vi "read from wavemeter_PB.vi"(2 "error in (no error)":errorcluster, 3 "Single Measurement?":bool=TRUE, 4 "Select Port":refnum<visa-resource-name>="COM1") -> (0 "error out":errorcluster={"status"=FALSE, "code"=1073676294, "source"="VISA Read in read from wavemeter.vi"}, 1 "frequency":string, 5 "Units":string)   [LabVIEW 2013]
uses:
  <vilib>/Instr/_visa.llb/VISA Configure Serial Port (Instr).vi
panel:
  in  "Case Constant\n(See Context Help)":bool
  in  "Tab Control":enum32{"Wavelength Monitor", "Nuts and Bolts"}(tab)=enum."Nuts and Bolts"
  out "Wavelength":string
  in  "Write Hex Command":string
  out "Array":dbl[](array[numeric])=[713.089] format="%.4f"
  out "return count":u32=7
  out "Wavemeter Front Panel Values":T1={"Quantity"="000713.089 nm", "Uncertainty is:"="LOW", "Averaging ON?"=FALSE, "Resolution:"="FIXED"}
  out "Array of buffer outputs":string[](array[string])=["+000713.089,2649,0200\r\n"]
  out "Buffer output":string="+000713.089,2649,0200\r\n"
  # "For Magnesium, port is \"COM1\".\nOn other computers, check Measurement\nand Automation Expolorer to see which\nRS-232 ports exist."
  # "This is quantity passed to calling VI."
  # "Make sure RS232 cable is plugged into\nsecond COM port (COM2) on back of \nBarium.  If you want to use COM1, you\nneed to change it on the back panel of\nthis VI."
  # "Writing commands to wavemeter does \nnot currently work.  Still in the trouble-\nshooting process.  Read will work fine."
  # "This stuff down here not useful for normal use.  Here \nfor trouble-shooting.  Feel free to ignore."
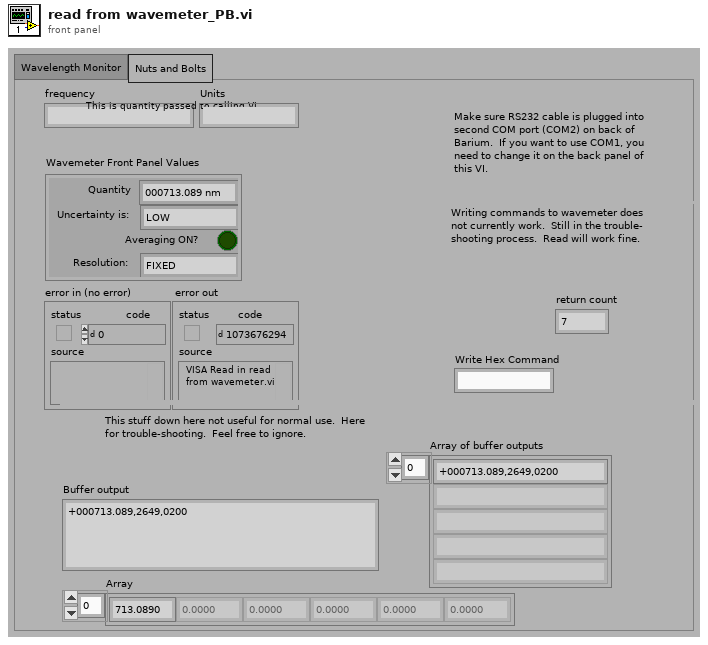
[diagram p1: front panel]
types:
  T1 = cluster{"Quantity":string, "Uncertainty is:":string, "Averaging ON?":bool, "Resolution:":string}
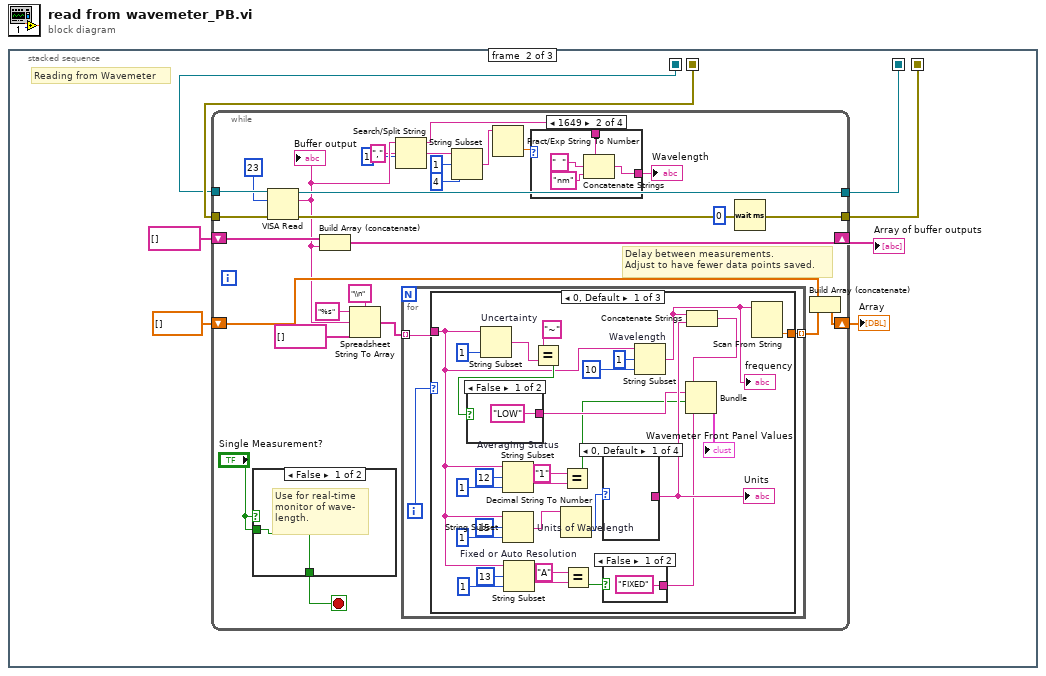
[diagram p0: block diagram]
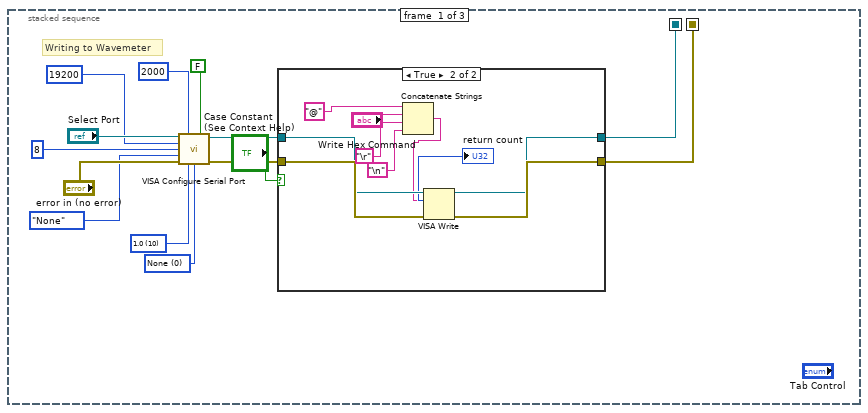
[diagram p2: hidden frame]
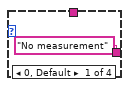
[diagram p4: hidden frame]
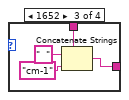
[diagram p5: hidden frame]
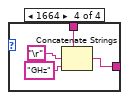
[diagram p6: hidden frame]
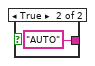
[diagram p8: hidden frame]
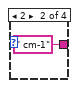
[diagram p9: hidden frame]
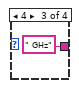
[diagram p10: hidden frame]
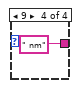
[diagram p11: hidden frame]
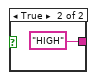
[diagram p12: hidden frame]
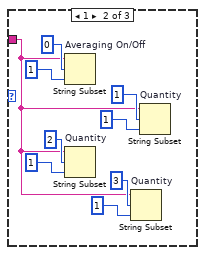
[diagram p13: hidden frame]
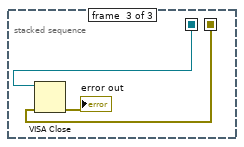
[diagram p15: hidden frame]
diagram:
  n1 = stacked-sequence {
    seq-local: [w12 _ _] -> [_ w33 _]
    seq-local: [w13 _ _] -> [_ w34 _]
    seq-local: [_ w31 _] -> [_ _ w125]
    seq-local: [_ w32 _] -> [_ _ w124]
    frame #0 {
      w1 = u16 0 items=["None"=0, "XON/XOFF"=1, "RTS/CTS"=2, "DTR/DSR"=4] ("flow control (0:none)")
      w2 = u16 10 items=["1.0"=10, "1.5"=15, "2.0"=20] ("stop bits (10: 1 bit)")
      # "Writing to Wavemeter"
      n2 = call-poly "VISA Configure Serial Port"("VISA resource name"="Select Port", "timeout (10sec)"=u32 2000, "Enable Termination\nChar (T)"=FALSE ("Enable Termination\nChar (T)"), "baud rate (9600)"=u32 19200, "data bits (8)"=u16 8, "parity (0:none)"=enum16{"None", "Odd", "Even", "Mark", "Space"}."None", "error in (no error)"="error in (no error)", "stop bits (10: 1 bit)"=w2, "flow control (0:none)"=w1) -> ("VISA resource name out"=w11:refnum<visa-resource-name>, "error out"=w14:errorcluster)  [unwired: 5 in]
      n3 = case shown="True" "Case Constant\n(See Context Help)" {
        tunnel: w14 -> [w15 w26]
        tunnel: [w15 w25] -> w13
        tunnel: [w16 w24] -> w12
        tunnel: w11 -> [w16 w23]
        frame False {
        }
        frame True {
          n4 = Concatenate Strings("@", "Write Hex Command", "\r", "\n") -> (w17:string)
          n5 = VISA Write(VISA resource name=w23, write buffer=w17, error in (no error)=w26) -> (VISA resource name out=w24:refnum<visa-resource-name>, return count=→"return count":u32, error out=w25:errorcluster)
        }
      }
    }
    frame #1 {
      # "Reading from Wavemeter"
      n6 = while {
        tunnel: w33 -> [w61]
        tunnel: w34 -> [w60]
        tunnel: [w58] -> w32
        tunnel: [w57] -> w31
        shift-right: [w56] -> w29
        shift-left: string[] [] -> [w55]
        shift-right: [w49] -> w27
        shift-left: dbl[] [] -> [w48]
        stop <- w46 stop-if-true
        # "Delay between measurements.\nAdjust to have fewer data points saved."
        n7 = case shown="False" "Single Measurement?" {
          tunnel: [w75 w76] -> w46
          tunnel: "Single Measurement?" -> [w75 w76]
          frame False {
            # "Use for real-time\nmonitor of wave-\nlength."
          }
          frame True {
            # "Stop loop after one\nmeasurement.  Used\nfor recording from PB."
          }
        }
        n8 = VISA Read(VISA resource name=w61, byte count=u32 23 ("byte count (0)"), error in (no error)=w60) -> (VISA resource name out=w57:refnum<visa-resource-name>, read buffer=w45:string, error out=w58:errorcluster)  [unwired: 1 out]
        "Buffer output" <- w45
        n9 = Build Array (concatenate)(w55, w45) -> (w56:string[])
        n10 = Spreadsheet String To Array(delimiter (Tab)="\\n", format string="%s", spreadsheet string=w45, array type (2D Dbl)=string[] []) -> (array=w50:string[])
        n11 = Search/Split String(string=w45, search string/char (-)=",", offset (0)=1) -> (substring before match=w37:string, match + rest of string=w42:string)  [unwired: 1 out]
        n12 = for {
          tunnel: w50 -> [w78] mode=indexing
          tunnel: [w77] -> w47 mode=indexing
          i -> [w79]
          n13 = case shown="0, Default" w79 {
            tunnel: w78 -> [w85 w115 _]
            tunnel: [w82 _ _] -> w77
            frame 0, Default {
              n14 = String Subset "Uncertainty"(string=w85, length (rest)=1 ("length (rest)")) -> (substring=w105:string)  [unwired: 1 in]
              n15 = String Subset "Averaging Status"(string=w85, offset (0)=12, length (rest)=1 ("length (rest)")) -> (substring=w101:string)
              n16 = String Subset "Units of Wavelength"(string=w85, offset (0)=15, length (rest)=1 ("length (rest)")) -> (substring=w97:string)
              n17 = String Subset "Fixed or Auto Resolution"(string=w85, offset (0)=13, length (rest)=1 ("length (rest)")) -> (substring=w87:string)
              n18 = Equal?(x="~", y=w105) -> (x = y?=w107:bool)
              n19 = case shown="False" w107 {
                tunnel: ["LOW" "HIGH"] -> w92
                frame False {
                }
                frame True {
                }
              }
              n20 = Decimal String To Number(string=w97) -> (number=w96:i32)  [unwired: 2 in, 1 out]
              n21 = Equal?(x="1", y=w101) -> (x = y?=w91:bool)
              n22 = Equal?(x="A", y=w87) -> (x = y?=w84:bool)
              n23 = case shown="0, Default" w96 {
                tunnel: [_ " cm-1" " GHz" " nm"] -> w93
                frame 0, Default {
                }
                frame 2 {
                }
                frame 4 {
                }
                frame 9 {
                }
              }
              "Units" <- w93
              n24 = case shown="False" w84 {
                tunnel: ["FIXED" "AUTO"] -> w83
                frame False {
                }
                frame True {
                }
              }
              n25 = String Subset "Wavelength"(string=w85, offset (0)=1, length (rest)=10 ("length (rest)")) -> (substring=w80:string)
              "frequency" <- w80
              n26 = Concatenate Strings(w80, w93) -> (w81:string)
              n27 = Bundle(w81, w92, w91, w83) -> (→"Wavemeter Front Panel Values":cluster{string, string, bool, string})  [unwired: 1 in]
              n28 = Scan From String(input string=w80) -> (output 1=w82:dbl)  [unwired: 4 in, 3 out]
            }
            frame 1 {
              n29 = String Subset "Averaging On/Off"(string=w115, offset (0)=0, length (rest)=1 ("length (rest)")) -> ()  [unwired: 1 out]
              n30 = String Subset "Quantity"(string=w115, offset (0)=2, length (rest)=1 ("length (rest)")) -> ()  [unwired: 1 out]
              n31 = String Subset "Quantity"(string=w115, offset (0)=3, length (rest)=1 ("length (rest)")) -> ()  [unwired: 1 out]
              n32 = String Subset "Quantity"(string=w115, offset (0)=1, length (rest)=1 ("length (rest)")) -> ()  [unwired: 1 out]
            }
            frame 2 {
            }
          }
        }
        n33 = String Subset(string=w42, offset (0)=1, length (rest)=4 ("length (rest)")) -> (substring=w38:string)
        n34 = Fract/Exp String To Number(string=w38) -> (number=w39:dbl)  [unwired: 3 in, 1 out]
        n35 = case shown="1649" w39 {
          tunnel: w37 -> [_ w66 w70 w74]
          tunnel: ["No measurement" w65 w69 w73] -> w36
          frame 0, Default {
          }
          frame 1649 {
            n36 = Concatenate Strings(w66, "  ", "nm" ("string")) -> (w65:string)
          }
          frame 1652 {
            n37 = Concatenate Strings(w70, "  " ("string"), "cm-1" ("string")) -> (w69:string)
          }
          frame 1664 {
            n38 = Concatenate Strings(w74, "\r", "GHz" ("string")) -> (w73:string)
          }
        }
        "Wavelength" <- w36
        n39 = Wait (ms)(milliseconds to wait=u32 0) -> ()  [unwired: 1 out]
        n40 = Build Array (concatenate)(w48, w47) -> (w49:dbl[])
      }
      "Array of buffer outputs" <- w29
      "Array" <- w27
    }
    frame #2 {
      n41 = VISA Close(VISA resource name=w125, error in (no error)=w124) -> (error out=→"error out":errorcluster)
    }
  }
